vi "sub_selectRandomIndex.vi"(11 "indexes":i32[](array[numeric])) -> (3 "random selected index":i32)   [LabVIEW 2018]
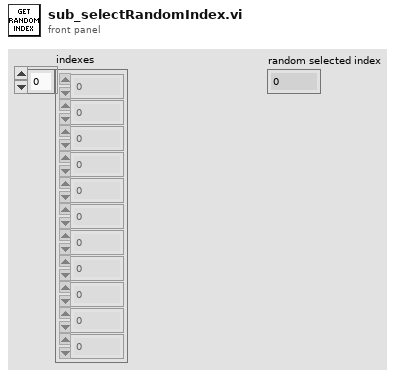
[diagram p1: front panel]
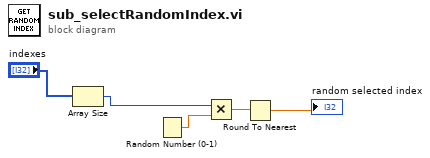
[diagram p0: block diagram]
diagram:
  n1 = Array Size(array="indexes") -> (size(s)=w4:i32)
  n2 = Random Number (0-1)() -> (number: 0 to 1=w3:dbl)
  n3 = Multiply(x=w4, y=w3) -> (x*y=w2:dbl)
  n4 = Round To Nearest(number=w2) -> (nearest integer value=→"random selected index":dbl)
